vi "PDF Details.vi"(0 "PDF Report IN":refnum<class "PDF Report Class.lvclass">, 7 "PDF Details":T1, 11 "error in (no error)":errorcluster) -> (4 "PDF Report OUT":refnum<class "PDF Report Class.lvclass">, 15 "error out":errorcluster)   [LabVIEW 2019, in "Exaprom PDF.lvlib"]
doc: "Write some metadatas to the PDF file:\n- Title\n- Subject\n- Keyword\n- Author\n- Creator\n\nVersion 1.0\nDeveloped by Jean-Marc Simard\nCopyright © 2010, Exaprom Inc.\nAll rights reserved.\nLicense: BSD\n\nWith iTextSharp 4.1.6 (http://itextsharp.sourceforge.net)\nunder Mozilla Public License Version 1.1\n(http://www.mozilla.org/MPL/MPL-1.1.html)"
uses:
  Controls/Initialization Controls/PDF Details.ctl
  LV Class/PDF Report Class/PDF Report Class.lvclass
  C:/work/niobrara_lv/labview pdf writer fixing/DLL/itextsharp.dll
  DLL/itextsharp.dll
  Exaprom PDF.lvlib
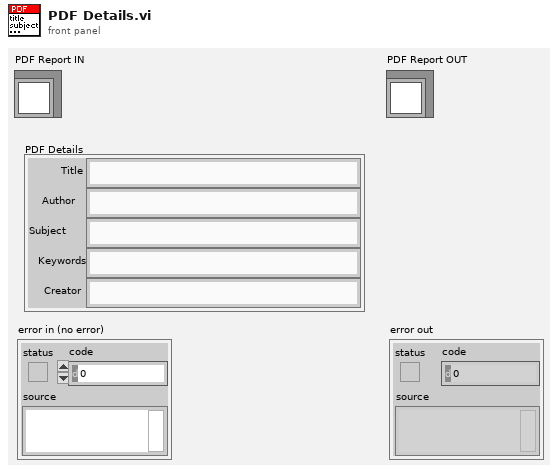
[diagram p1: front panel]
types:
  T1 = typedef "Exaprom PDF.lvlib/PDF Details.ctl" = cluster{"Title":string, "Author":string, "Subject":string, "Keywords":string, "Creator":string}
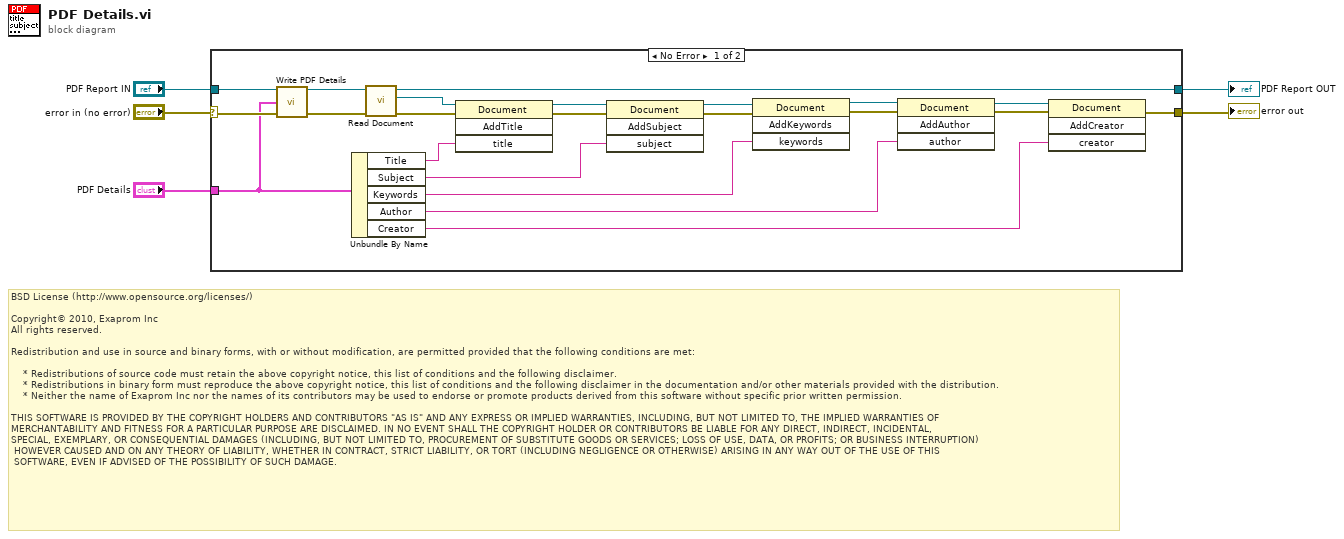
[diagram p0: block diagram]
diagram:
  # "BSD License (http://www.opensource.org/licenses/)\n\nCopyright© 2010, Exaprom Inc\nAll rights reserved.\n\nRedistribution and use in source and binary forms, with or without modification, are permitted provided that the following conditions are met:\n\n    * Redistributions of source code must retain the above copyright notice, this list of conditions and the following disclaimer.\n    * Redistributions in binary form must reproduce the above copyright notice, this list of conditions and the following disclaimer in the documentation and/or other materials provided with the distribution.\n    * Neither the name of Exaprom Inc nor the names of its contributors may be used to endorse or promote products derived from this software without specific prior written permission.\n\nTHIS SOFTWARE IS PROVIDED BY THE COPYRIGHT HOLDERS AND CONTRIBUTORS \"AS IS\" AND ANY EXPRESS OR IMPLIED WARRANTIES, INCLUDING, BUT NOT LIMITED TO, THE IMPLIED WARRANTIES OF \nMERCHANTABILITY AND FITNESS FOR A PARTICULAR PURPOSE ARE DISCLAIMED. IN NO EVENT SHALL THE COPYRIGHT HOLDER OR CONTRIBUTORS BE LIABLE FOR ANY DIRECT, INDIRECT, INCIDENTAL,\nSPECIAL, EXEMPLARY, OR CONSEQUENTIAL DAMAGES (INCLUDING, BUT NOT LIMITED TO, PROCUREMENT OF SUBSTITUTE GOODS OR SERVICES; LOSS OF USE, DATA, OR PROFITS; OR BUSINESS INTERRUPTION)\n HOWEVER CAUSED AND ON ANY THEORY OF LIABILITY, WHETHER IN CONTRACT, STRICT LIABILITY, OR TORT (INCLUDING NEGLIGENCE OR OTHERWISE) ARISING IN ANY WAY OUT OF THE USE OF THIS\n SOFTWARE, EVEN IF ADVISED OF THE POSSIBILITY OF SUCH DAMAGE."
  n1 = case shown="No Error" "error in (no error)" {
    selector: "error in (no error)" -> [w12 w28]
    tunnel: "PDF Details" -> [w6 _]
    tunnel: [w18 w28] -> w4
    tunnel: "PDF Report IN" -> [w9 w27]
    tunnel: [w8 w27] -> w1
    frame No Error {
      n2 = call-dynamic "Write PDF Details.vi"("PDF Report Class in"=w9, "PDF Details"=w6) -> ("PDF Report Class out"=w7:refnum<class "PDF Report Class.lvclass">)  [unwired: 12 in, 1 out]
      n3 = Unbundle By Name(w6) -> ("Title"=w13:string, "Subject"=w17:string, "Keywords"=w16:string, "Author"=w15:string, "Creator"=w14:string)
      n4 = call-dynamic "Read Document.vi"("error in (no error)"=w12, "PDF Report Class in"=w7) -> ("error out"=w11:errorcluster, "Document"=w10:refnum<k24>, "PDF Report Class out"=w8:refnum<class "PDF Report Class.lvclass">)  [unwired: 7 in]
      n5 = invoke class="Document" method="AddTitle"(reference=w10, error in=w11, "title"=w13) -> (reference out=w26:refnum<k24>, error out=w25:errorcluster)  [unwired: 1 in, 2 out]
      n6 = invoke class="Document" method="AddSubject"(reference=w26, error in=w25, "subject"=w17) -> (reference out=w24:refnum<k24>, error out=w23:errorcluster)  [unwired: 1 in, 2 out]
      n7 = invoke class="Document" method="AddKeywords"(reference=w24, error in=w23, "keywords"=w16) -> (reference out=w22:refnum<k24>, error out=w21:errorcluster)  [unwired: 1 in, 2 out]
      n8 = invoke class="Document" method="AddAuthor"(reference=w22, error in=w21, "author"=w15) -> (reference out=w19:refnum<k24>, error out=w20:errorcluster)  [unwired: 1 in, 2 out]
      n9 = invoke class="Document" method="AddCreator"(reference=w19, error in=w20, "creator"=w14) -> (error out=w18:errorcluster)  [unwired: 1 in, 3 out]
    }
    frame Error {
    }
  }
  "error out" <- w4
  "PDF Report OUT" <- w1
